vi "Resize Window.vi"(6 "Variant in":variant, 7 "Shift Pressed?":bool, 8 "error in (no error)":errorcluster, 10 "QD Combo Box Ref":refnum<vi>, 11 "QD Launch VI Ref":refnum<vi>) -> (0 "error out":errorcluster, 4 "Variant out":variant)   [LabVIEW 2019]
doc: "Resizes the front panel or block diagram window to the content bounds. The front panel will also reset the panel origins to 0, 0 and adjusts for the Minimum Window Size property.\n\nCreated by: Ryan Pacini\n\nDefault Shortcut - [E]"
uses:
  _Script/support/Script.lvlib
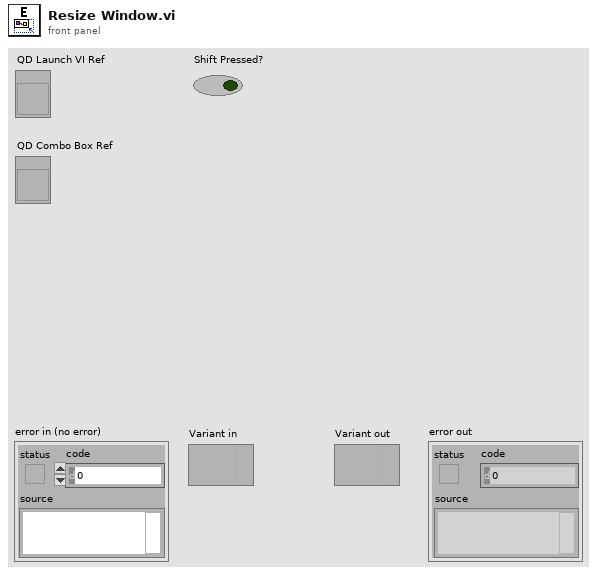
[diagram p1: front panel]
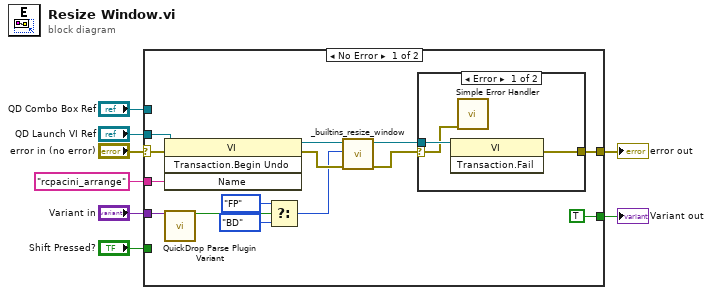
[diagram p0: block diagram]
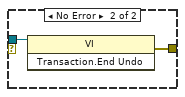
[diagram p2: hidden frame]
diagram:
  n1 = case shown="No Error" "error in (no error)" {
    selector: "error in (no error)" -> [w22 w28]
    tunnel: [w21 w28] -> w3
    tunnel: "QD Launch VI Ref" -> [w17 _]
    tunnel: "rcpacini_arrange" ("Undo Name") -> [w20 _]
    tunnel: "Variant in" -> [w18 _]
    tunnel: [TRUE _] -> w4
    tunnel: "QD Combo Box Ref" -> [_ _]
    tunnel: "Shift Pressed?" -> [_ _]
    frame No Error {
      n2 = invoke class="VI" method="Transaction.Begin Undo"(reference=w17, error in=w22, "Name"=w20) -> (reference out=w16:refnum<vi>, error out=w15:errorcluster)  [unwired: 1 in, 2 out]
      n3 = call <vilib>:"QuickDrop Parse Plugin Variant.vi"("QDKS Variant in"=w18) -> ("QD Launch VI Panel?"=w12:bool)  [unwired: 12 in, 2 out]
      n4 = Select(t=enum8{"FP", "BD"}."FP" ("Panel"), s=w12, f=enum8{"FP", "BD"}."BD" ("Panel")) -> (s? t:f=w9:enum8{"FP", "BD"})
      n5 = call "_builtins_resize_window.vi"("error in (no error)"=w15, "Focus"=w9, "VI Refnum in"=w16) -> ("error out"=w10:errorcluster, "VI Refnum out"=w11:refnum<vi>)  [unwired: 7 in]
      n6 = case shown="Error" w10 {
        selector: w10 -> [w23 _]
        tunnel: w11 -> [w24 w26]
        tunnel: [w25 w27] -> w21
        frame Error {
          n7 = invoke class="VI" method="Transaction.Fail"(reference=w24) -> (error out=w25:errorcluster)  [unwired: 2 in, 2 out]
          n8 = call <vilib>:"Simple Error Handler.vi"("error in (no error)"=w23) -> ()  [unwired: 4 in, 5 out]
        }
        frame No Error {
          n9 = invoke class="VI" method="Transaction.End Undo"(reference=w26) -> (error out=w27:errorcluster)  [unwired: 2 in, 2 out]
        }
      }
    }
    frame Error {
    }
  }
  "error out" <- w3
  "Variant out" <- w4
